vi "接收解析.vi"(15 "data in":string) -> (0 "内容说明":string, 1 "内容标识":string, 2 "时标":string, 3 "帧头":string, 4 "重算CRC32":string, 5 "帧数":string, 7 "帧号":string, 8 "data out":string, 9 "帧长":string, 10 "CRC":string, 11 "帧内容":string, 13 "结束标志":string)   [LabVIEW 2016, in "数据传输系统-05.lvlib" / "自动更新.lvlib" / "TCP文件传输系统.lvlib" / "TCP接收文件.lvlib"]
panel:
  out "长度":i32
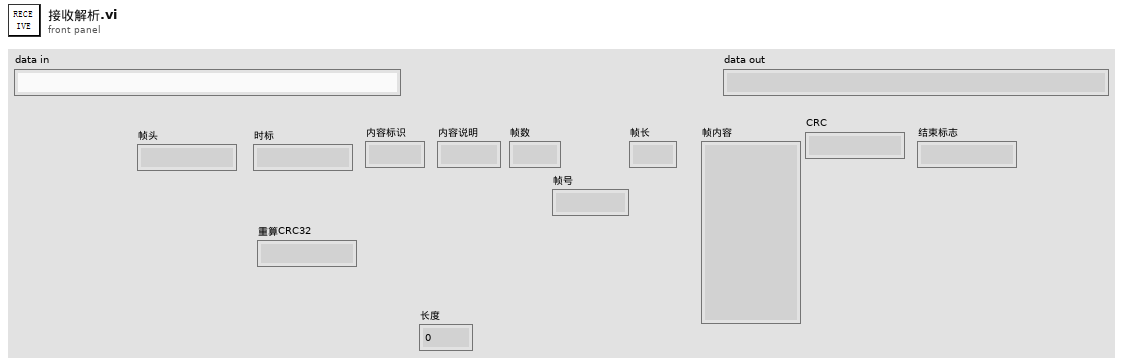
[diagram p1: front panel]
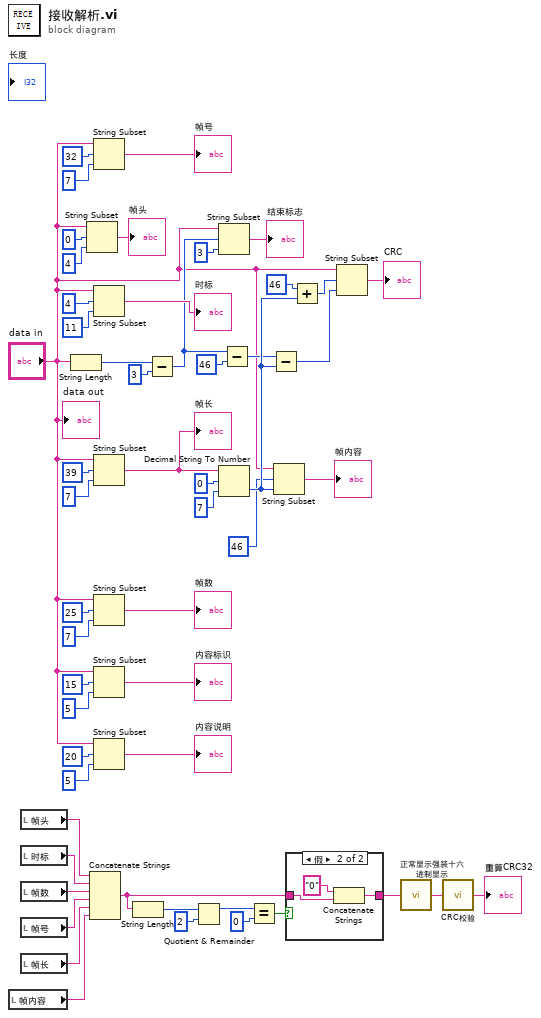
[diagram p0: block diagram]
diagram:
  n1 = local read "帧内容"() -> (w10:string)
  n2 = local read "帧头"() -> (w15:string)
  n3 = local read "时标"() -> (w14:string)
  n4 = local read "帧数"() -> (w13:string)
  n5 = local read "帧号"() -> (w12:string)
  n6 = local read "帧长"() -> (w11:string)
  n7 = String Length(string="data in") -> (length=w51:i32)
  n8 = String Subset(string="data in", offset (0)=0 ("偏移量(0)"), length (rest)=4 ("长度（剩余）")) -> (substring=→"帧头":string)
  n9 = Concatenate Strings(w15, w14, w13, w12, w11, w10) -> (w7:string)
  n10 = String Subset(string="data in", offset (0)=32 ("偏移量(0)"), length (rest)=7 ("长度（剩余）")) -> (substring=→"帧号":string)
  n11 = String Subset(string="data in", offset (0)=4 ("偏移量(0)"), length (rest)=11 ("长度（剩余）")) -> (substring=→"时标":string)
  n12 = String Subset(string="data in", offset (0)=39 ("偏移量(0)"), length (rest)=7 ("长度（剩余）")) -> (substring=w43:string)
  "帧长" <- w43
  n13 = String Subset(string="data in", offset (0)=25 ("偏移量(0)"), length (rest)=7 ("长度（剩余）")) -> (substring=→"帧数":string)
  n14 = String Subset(string="data in", offset (0)=15 ("偏移量(0)"), length (rest)=5 ("长度（剩余）")) -> (substring=→"内容标识":string)
  n15 = String Subset(string="data in", offset (0)=20 ("偏移量(0)"), length (rest)=5 ("长度（剩余）")) -> (substring=→"内容说明":string)
  n16 = String Length(string=w7) -> (length=w9:i32)
  n17 = Subtract(x=w51, y=3) -> (x-y=w21:i32)
  n18 = Quotient & Remainder(x=w9, y=2) -> (x-y*floor(x/y)=w3:i32)  [unwired: 1 out]
  n19 = String Subset(string="data in", offset (0)=w21, length (rest)=3 ("长度（剩余）")) -> (substring=→"结束标志":string)
  n20 = Decimal String To Number(string=w43, offset=0 ("偏移量"), default (0L)=7 ("默认(0 I32)")) -> (number=w49:i32)  [unwired: 1 out]
  n21 = Subtract(x=w21, y=46) -> (x-y=w46:i32)
  n22 = Equal?(x=w3, y=0) -> (x = y?=w1:bool)
  n23 = Subtract(x=w46, y=w49) -> (x-y=w19:i32)
  n24 = String Subset(string="data in", offset (0)=46 ("偏移量(0)"), length (rest)=w49) -> (substring=→"帧内容":string)
  n25 = case shown="假" w1 {
    tunnel: w7 -> [w54 w56]
    tunnel: [w54 w55] -> w6
    frame True {
    }
    frame False {
      n26 = Concatenate Strings("0" ("字符串"), w56) -> (w55:string)
    }
  }
  n27 = Add(x=46 ("偏移量(0)"), y=w49) -> (x+y=w20:i32)
  n28 = String Subset(string="data in", offset (0)=w20, length (rest)=w19) -> (substring=→"CRC":string)
  n29 = call "正常显示强装十六进制显示.vi"("正常格式显示字符串"=w6) -> ("十六进制格式显示"=w5:string)
  n30 = call "CRC校验.vi"("要校验的字符串（十六进制显示）"=w5) -> ("CRC32效验码输出"=→"重算CRC32":string)
  "data out" <- "data in"
